vi "Example Colour JSON items in a string control.vi"() -> ()   [LabVIEW 2015]
uses:
  JSONtext.lvlib
panel:
  out "JSON 2":string
  in  "JSON":string="{\r        \"sequence\":22222222,\r        \"prev_out\":{\r          \"spent\":true,\r          \"tx_index\":99005469,\r          \"type\":1,\r          \"addr\":\"Blah Blah Blah\",\r          \"value\":1,\r          \"n\":0,\r          \"script\":\"76a91477f4c9ee75e449a74c21a4decfb50519cbc245b388ac\"\r        }"
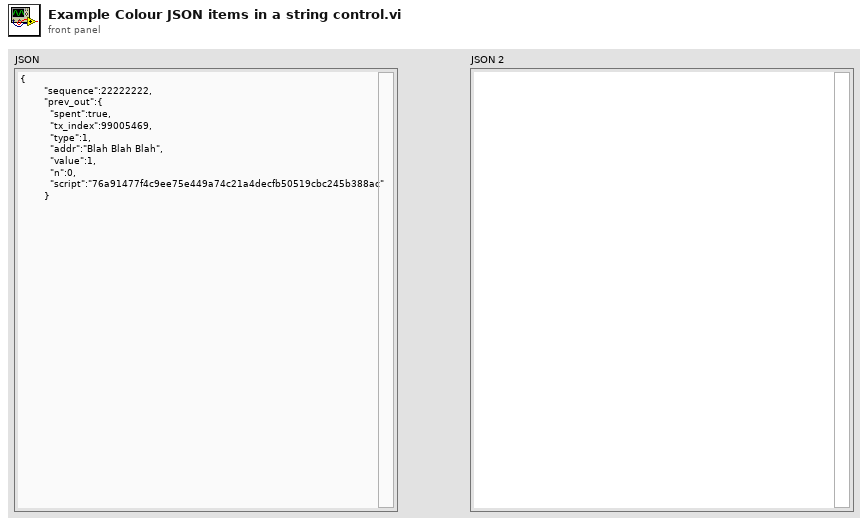
[diagram p1: front panel]
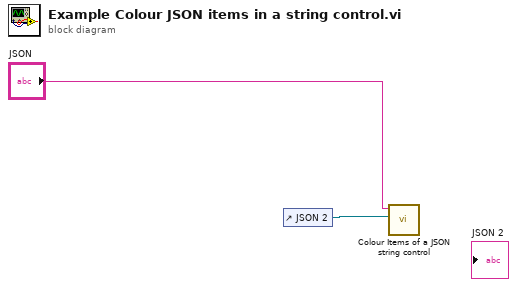
[diagram p0: block diagram]
diagram:
  n1 = control-ref of="JSON 2"() -> (w2:refnum<vi>)
  n2 = call "Colour Items of a JSON string control.vi"("String Control"=w2, "JSON"="JSON") -> ()  [unwired: 10 in]
